vi "instance count allowed.vi"(8 "error in":errorcluster, 11 "Increment configuration in":refnum<class "Increment configuration.lvclass">) -> (0 "error out":errorcluster, 2 "instances allowed":i32, 3 "Increment configuration out":refnum<class "Increment configuration.lvclass">)   [LabVIEW 2015, in "Increment configuration.lvclass"]
uses:
  Increment configuration.lvclass
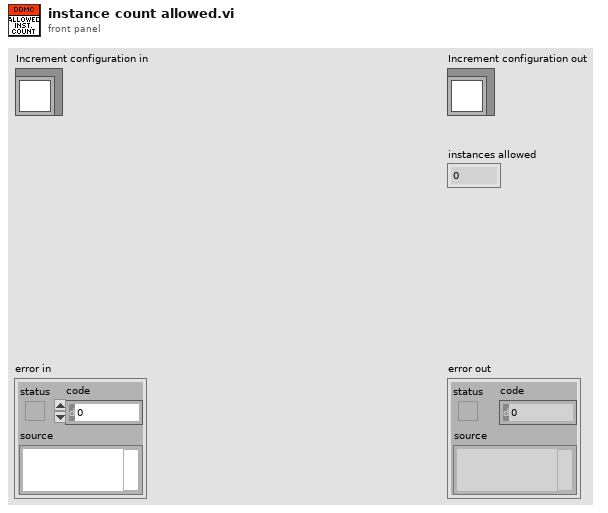
[diagram p1: front panel]
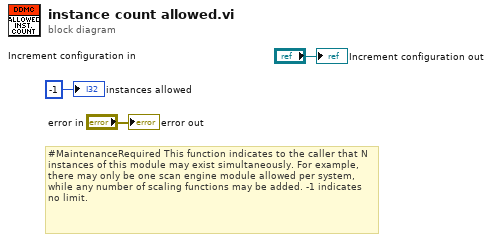
[diagram p0: block diagram]
diagram:
  # "#MaintenanceRequired This function indicates to the caller that N instances of this module may exist simultaneously. For example, there may only be one scan engine module allowed per system, while any number of scaling functions may be added. -1 indicates no limit."
  "error out" <- "error in"
  "Increment configuration out" <- "Increment configuration in"
  "instances allowed" <- -1 ("instances allowed")
